vi "ProdaNG.CreateProcessStepResult.vi"(8 "error in (no error)":errorcluster, 9 "ProcessStepResult":T1, 10 "ID":T2, 11 "dbHandle":i32) -> (0 "error out":errorcluster, 1 "ProcessStepResult 2":T1, 3 "dbHandle out":i32)   [LabVIEW 2016]
doc: "This function returns a product structure for a product, which is identified by a part and a serial number.\nImportant information: The field 'individual' was taken over from the field 'allgemein' of the legacy data directly. Because of this most products have the value 0 further on and only a few the value 1. \nParameter:\nhandle is an Integer, which is returned by the function Login() at the creation of a new connection.\nwabcoPartId is the Id of the part.\nserialNumber is the serial number of the product for the part above.\nproduct is a pointer on a product structure, which is filled if the returncode is 0. The structure must be defined in the calling program.\n\nReturncodes:\n0 No error\n< 0 ORACLE Error code\n6 (ERROR_INVALID_HANDLE) in case of an invalid handle\n1403 Record does not exist"
uses:
  Controls/ProdaNG.ProcessStepResult.ctl
  Controls/ProdaNG.Identification.ctl
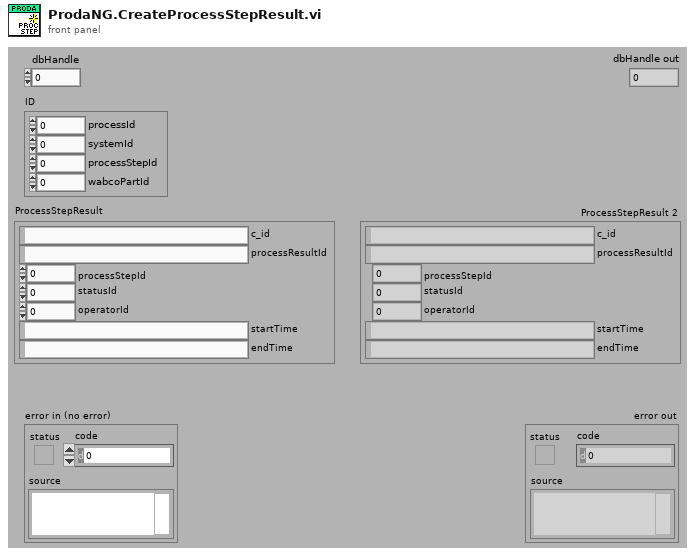
[diagram p1: front panel]
types:
  T1 = typedef "ProdaNG.ProcessStepResult.ctl" = cluster{"c_id":string, "processResultId":string, "processStepId":i32, "statusId":i32, "operatorId":i32, "startTime":string, "endTime":string}
  T2 = typedef "ProdaNG.Identification.ctl" = cluster{"processId":i32, "systemId":i32, "processStepId":i32, "wabcoPartId":i32}
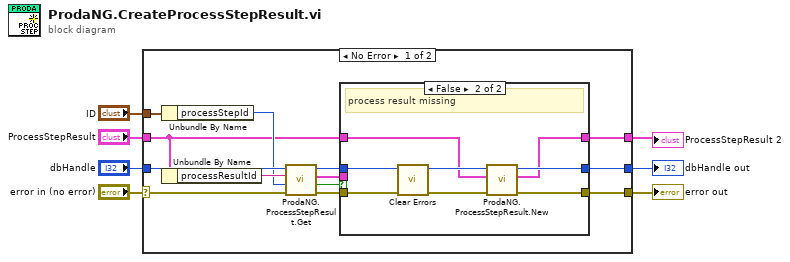
[diagram p0: block diagram]
diagram:
  n1 = case shown="No Error" "error in (no error)" {
    selector: "error in (no error)" -> [w14 w33]
    tunnel: [w12 w33] -> w6
    tunnel: "dbHandle" -> [w18 w32]
    tunnel: [w8 w32] -> w4
    tunnel: "ProcessStepResult" -> [w13 w31]
    tunnel: "ID" -> [w16 _]
    tunnel: [w11 w31] -> w1
    frame No Error {
      n2 = Unbundle By Name(w16) -> ("processStepId"=w15:i32)
      n3 = Unbundle By Name(w13) -> ("processResultId"=w20:string)
      n4 = call "ProdaNG.ProcessStepResult.Get.vi"("error in (no error)"=w14, "processStepId"=w15, "processResultId"=w20, "dbHandle"=w18) -> ("error out"=w9:errorcluster, "Found"=w10:bool, "ProcessStepResult"=w17:T1, "dbHandle out"=w19:i32)  [unwired: 4 in]
      n5 = case shown="False" w10 {
        tunnel: w19 -> [w23 w30]
        tunnel: [w23 w29] -> w8
        tunnel: w17 -> [w21 _]
        tunnel: w13 -> [_ w24]
        tunnel: [w22 w26] -> w12
        tunnel: [w21 w27] -> w11
        tunnel: w9 -> [w22 w25]
        frame True {
          # "process step result exists"
        }
        frame False {
          # "process result missing"
          n6 = call <vilib>:"Clear Errors.vi"("error in (no error)"=w25) -> ("error out"=w28:errorcluster)  [unwired: 5 in, 1 out]
          n7 = call "ProdaNG.ProcessStepResult.New.vi"("error in (no error)"=w28, "ProcessStepResult"=w24, "dbHandle"=w30) -> ("error out"=w26:errorcluster, "ProcessStepResult out"=w27:T1, "dbHandle"=w29:i32)  [unwired: 6 in]
        }
      }
    }
    frame Error {
    }
  }
  "error out" <- w6
  "dbHandle out" <- w4
  "ProcessStepResult 2" <- w1
